vi "Thev-Vectorize Data.vi"(7 "2D CDB":cdb[][](array[numeric])) -> (8 "1D DBL":dbl[](array[numeric]))   [LabVIEW 2015]
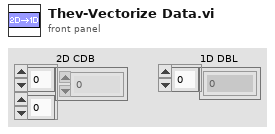
[diagram p1: front panel]
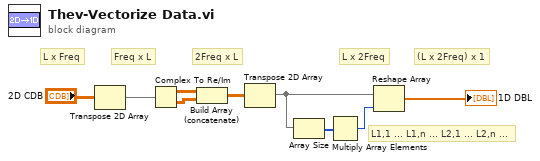
[diagram p0: block diagram]
diagram:
  # "L1,1 ... L1,n ... L2,1 ... L2,n ..."
  # "(L x 2Freq) x 1"
  # "L x 2Freq"
  # "2Freq x L"
  # "Freq x L"
  # "L x Freq"
  n1 = Transpose 2D Array(2D array="2D CDB") -> (transposed array=w8:cdb[][])
  n2 = Complex To Re/Im(x + iy=w8) -> (x=w7:dbl[][], y=w6:dbl[][])
  n3 = Build Array (concatenate)(w7, w6) -> (w5:dbl[][])
  n4 = Transpose 2D Array(2D array=w5) -> (transposed array=w3:dbl[][])
  n5 = Array Size(array=w3) -> (size(s)=w1:i32[])
  n6 = Multiply Array Elements(1:w1) -> (0:w2:i32)
  n7 = Reshape Array(w3, w2) -> (→"1D DBL":dbl[])
